vi "to string.vi"(8 "error in":errorcluster, 11 "tag bus configurable plugin module configuration in":refnum<class "tag bus processing plugin module configuration.lvclass">) -> (0 "error out":errorcluster, 1 "data":string, 2 "version":string, 3 "tag bus configurable plugin module configuration out":refnum<class "tag bus processing plugin module configuration.lvclass">)   [LabVIEW 2013, in "tag bus processing plugin module configuration.lvclass"]
doc: "Provides an interface for saving a module configuration to a file or other serialized data source. It is recommended that all children of this class store data in two sets--data required for its own initialization, and any data required for parent initialization--and that each implementation uses the <b>Call Parent Method</b> primitive to serialize parent information."
uses:
  tag bus processing plugin module configuration.lvclass
  <vilib>/NI/Tag Bus Module Framework/module configuration/TBM module configuration.lvclass
  tag bus processing plugin module configuration.lvclass/tag bus processing plugin module configuration.ctl
  current version.vi
  <vilib>/NI/Tag Bus Module Framework/channel/TBM channel.lvclass
  <vilib>/NI/Configuration Framework/serializable configuration/NISE_CEF_serializable configuration.lvclass
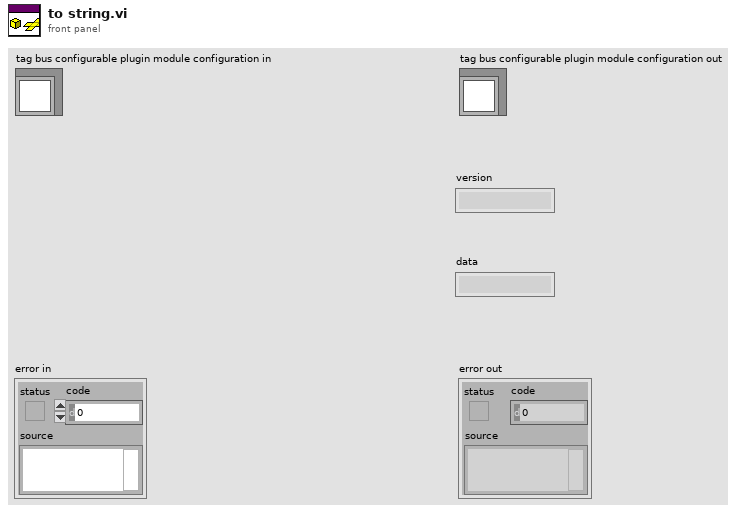
[diagram p1: front panel]
types:
  T1 = typedef "tag bus processing plugin module configuration.lvclass/processing channels.ctl" = cluster{"parameter":refnum<class "TBM channel.lvclass">, "result":refnum<class "TBM channel.lvclass">}
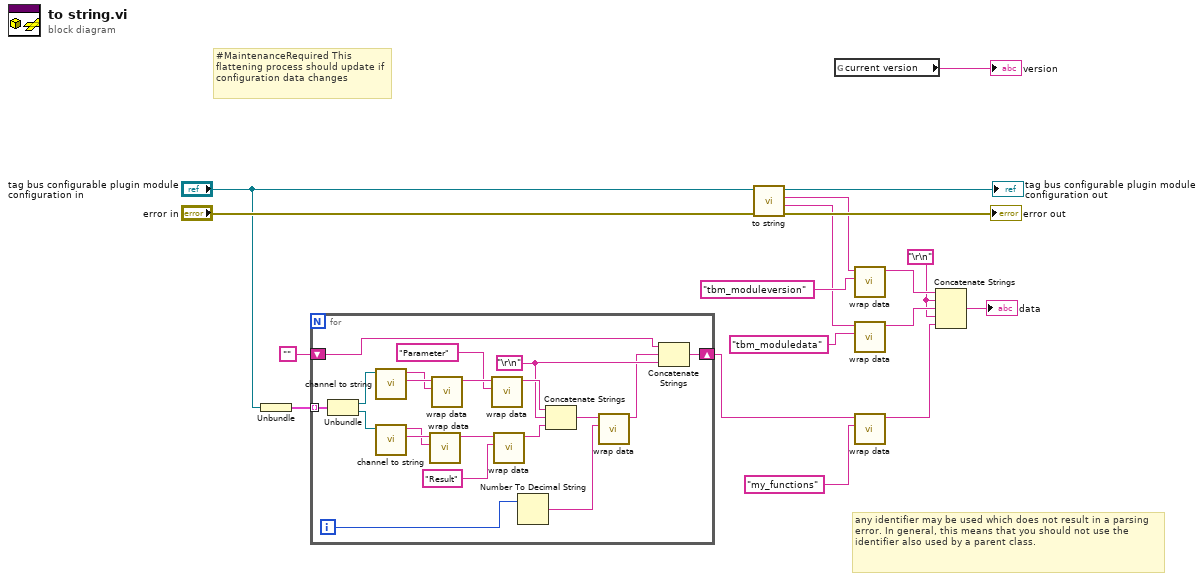
[diagram p0: block diagram]
diagram:
  w1 = "\r\n"
  # "any identifier may be used which does not result in a parsing error. In general, this means that you should not use the identifier also used by a parent class."
  # "#MaintenanceRequired This flattening process should update if configuration data changes"
  n1 = Unbundle("tag bus configurable plugin module configuration in") -> (w5:T1[])
  n2 = for {
    tunnel: w5 -> [w38] mode=indexing
    shift-right: [w25] -> w3
    shift-left: "" -> [w24]
    i -> [w22]
    w23 = "\r\n"
    n3 = Unbundle(w38) -> ("parameter"=w37:refnum<class "TBM channel.lvclass">, "result"=w36:refnum<class "TBM channel.lvclass">)
    n4 = call <vilib>:"channel to string.vi"("channel in"=w37) -> ("channel data"=w35:string, "identifier"=w32:string)  [unwired: 9 in]
    n5 = call <vilib>:"channel to string.vi"("channel in"=w36) -> ("channel data"=w34:string, "identifier"=w33:string)  [unwired: 9 in]
    n6 = call <vilib>:"wrap data.vi"("identifier"=w33, "data to wrap"=w34) -> ("wrapped data"=w29:string)  [unwired: 9 in]
    n7 = call <vilib>:"wrap data.vi"("identifier"=w32, "data to wrap"=w35) -> ("wrapped data"=w31:string)  [unwired: 9 in]
    n8 = call <vilib>:"wrap data.vi"("identifier"="Parameter", "data to wrap"=w31) -> ("wrapped data"=w27:string)  [unwired: 9 in]
    n9 = call <vilib>:"wrap data.vi"("identifier"="Result", "data to wrap"=w29) -> ("wrapped data"=w26:string)  [unwired: 9 in]
    n10 = Number To Decimal String(number=w22) -> (decimal integer string=w20:string)  [unwired: 1 in]
    n11 = Concatenate Strings(w27, w23, w26) -> (w21:string)
    n12 = call <vilib>:"wrap data.vi"("identifier"=w20, "data to wrap"=w21) -> ("wrapped data"=w19:string)  [unwired: 9 in]
    n13 = Concatenate Strings(w24, w19, w23) -> (w25:string)
  }
  n14 = call-parent "to string.vi"("error in"="error in", "module configuration in"="tag bus configurable plugin module configuration in") -> ("error out"=→"error out":errorcluster, "data"=w6:string, "version"=w7:string, "module configuration out"=→"tag bus configurable plugin module configuration out":refnum<class "tag bus processing plugin module configuration.lvclass">)  [unwired: 6 in]
  n15 = global read "current version.vi" "current version"() -> (→"version":string)
  n16 = call <vilib>:"wrap data.vi"("identifier"="tbm_moduleversion" ("additional identifier"), "data to wrap"=w7) -> ("wrapped data"=w12:string)  [unwired: 9 in]
  n17 = call <vilib>:"wrap data.vi"("identifier"="tbm_moduledata" ("additional identifier"), "data to wrap"=w6) -> ("wrapped data"=w11:string)  [unwired: 9 in]
  n18 = call <vilib>:"wrap data.vi"("identifier"="my_functions" ("additional identifier"), "data to wrap"=w3) -> ("wrapped data"=w2:string)  [unwired: 9 in]
  n19 = Concatenate Strings(w12, w1, w11, w1, w2) -> (→"data":string)
